vi "PixeLink OpenFocSpot.vi"(7 "Open Focal spot":path=path "G:/Développement de Programmes/Programmes/octo-labview/PixeLink - Homebrew/Data") -> ()   [LabVIEW 2014]
panel:
  in  "SOTP":bool
  out "Intensity (measured)\nx10^18 W/cm²":dbl=2.0
  out "Intensity (gaussian)\nx10^18 W/cm²":dbl=2.0
  out "Peak power (TW)":dbl=2.0
  out "FWHM y (µm)":dbl=2.0
  out "FWHM x (µm)":dbl=2.0
  in  "Transmission":dbl=0.5
  in  "Duration FWHM (fs)":dbl=4.5
  in  "Pulse Energy (mJ)":dbl=5.0
  in  "Calibration µm/px":dbl=0.5
  in  "Compute":bool
  out "Focal Spot":dbl[][](graph)
  out "Background":dbl[][](graph)
  out "ROI":dbl[][](graph)
  in  "Select Background":bool
  in  "Select ROI":bool
  # "SOTP"
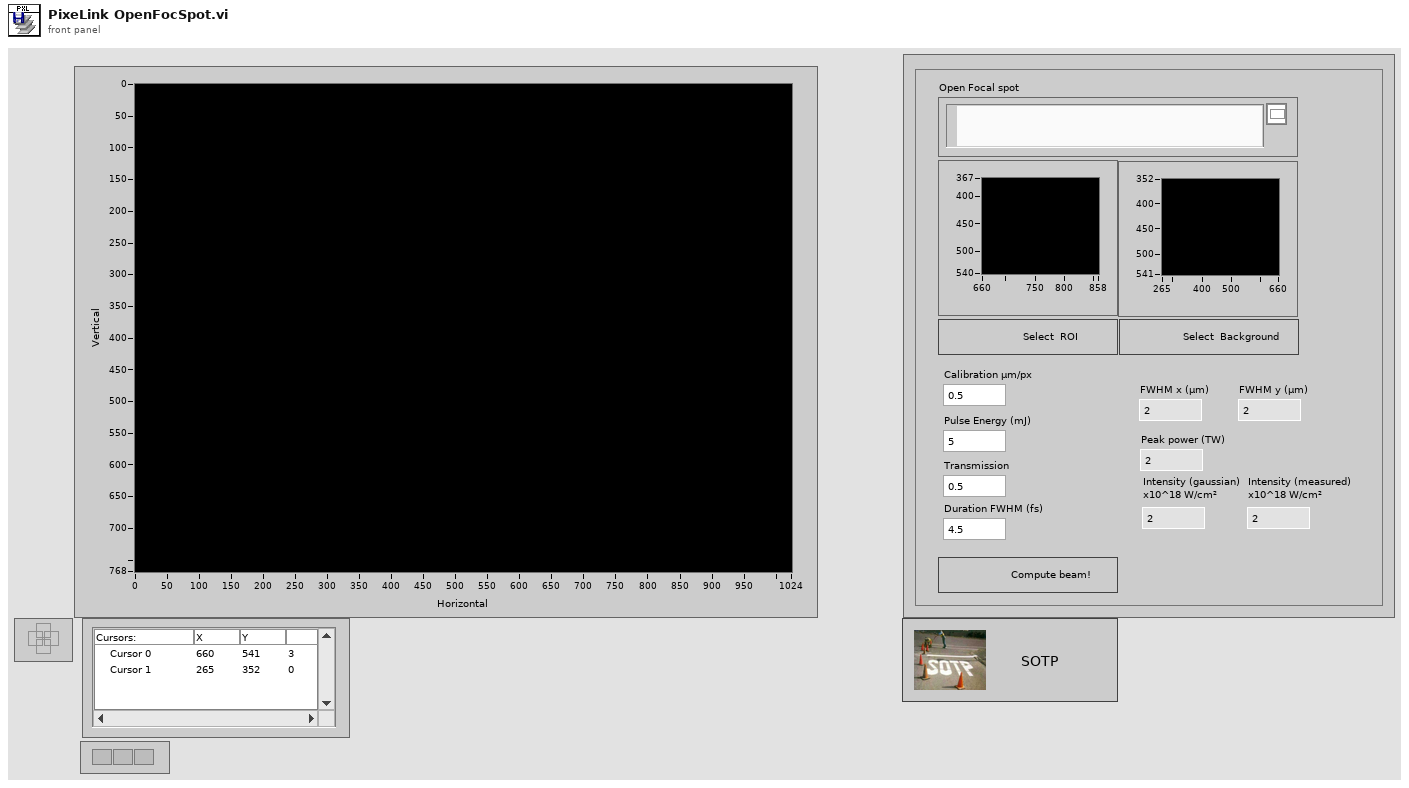
[diagram p1: front panel]
types:
  T1 = typedef "Image Type" = u32
  T2 = typedef "IMAQ Image.ctl" = refnum<image>
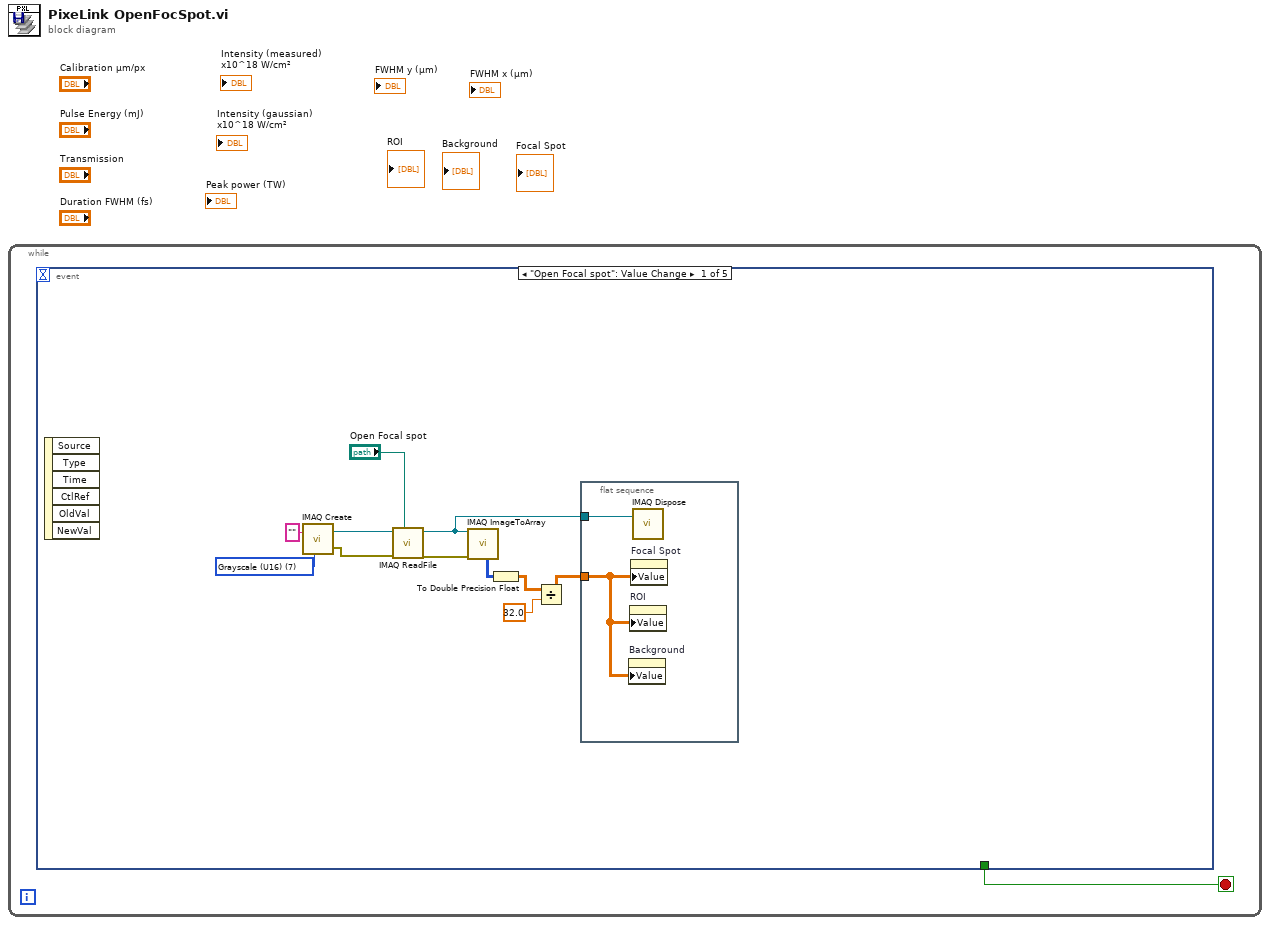
[diagram p0: block diagram]
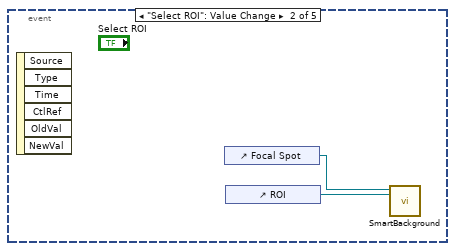
[diagram p2: hidden frame]
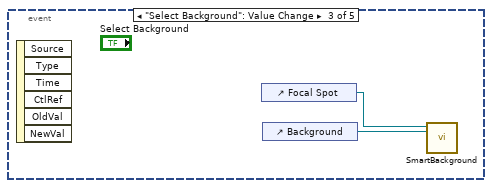
[diagram p3: hidden frame]
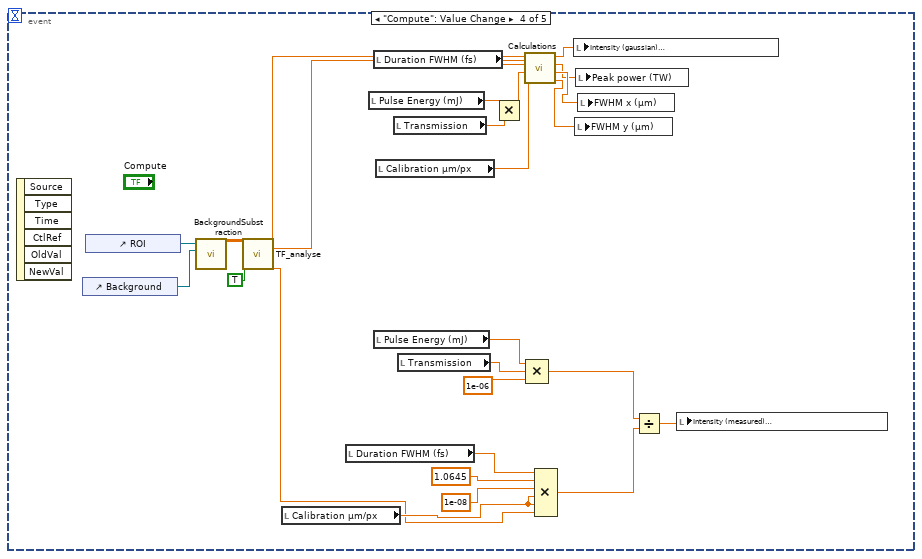
[diagram p4: hidden frame]
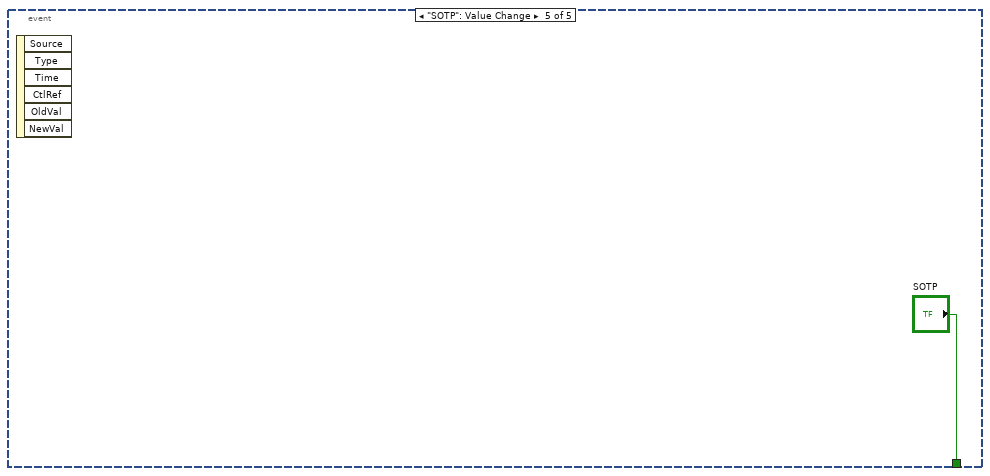
[diagram p5: hidden frame]
diagram:
  n1 = while {
    stop <- w1 stop-if-true
    n2 = event shown="[0] \"Open Focal spot\": Value Change" {
      selector: _ -> [_ _ _ _ _]
      dyn-events: _ -> [_ _ _ _ _]
      timeout: _ -> [_ _ _ _ _]
      tunnel: [_ _ _ _ "SOTP"] -> w1
      event "Open Focal spot": Value Change {
        w6 = T1 7 items=["Grayscale (U8)", "Grayscale (I16)", "Grayscale (SGL)", "Complex (CSG)", "RGB (U32)", "HSL (U32)", "RGB (U64)", "Grayscale (U16)"] ("Image Type")
        n3 = event-data() -> ()  [unwired: 1 in, 6 out]
        n4 = call "IMAQ Create"("Image Name"="", "Image Type"=w6) -> ("New Image"=w11:T2, "error out"=w9:errorcluster)  [unwired: 3 in]
        n5 = call "IMAQ ReadFile"("File Path"="Open Focal spot", "error in (no error)"=w9, "Image"=w11) -> ("error out"=w8:errorcluster, "Image Out"=w5:T2)  [unwired: 4 in, 3 out]
        n6 = call "IMAQ ImageToArray"("error in (no error)"=w8, "Image"=w5) -> ("Image Pixels (U16)"=w7:u16[][])  [unwired: 2 in, 4 out]
        n7 = To Double Precision Float(number=w7) -> (double precision float=w3:dbl[][])
        n8 = Divide(x=w3, y=32.0) -> (x/y=w4:dbl[][])
        n9 = flat-sequence {
          tunnel: w4 -> [w13]
          tunnel: w5 -> [w14]
          frame #0 {
            n10 = property on="Background" class="IntGraph (strict)"("Value"=w13) -> ()  [unwired: 2 in, 2 out]
            n11 = property on="ROI" class="IntGraph (strict)"("Value"=w13) -> ()  [unwired: 2 in, 2 out]
            n12 = property on="Focal Spot" class="IntGraph (strict)"("Value"=w13) -> ()  [unwired: 2 in, 2 out]
            n13 = call "IMAQ Dispose"("Image"=w14) -> ()  [unwired: 5 in, 1 out]
          }
        }
      }
      event "Select ROI": Value Change {
        n14 = event-data() -> ()  [unwired: 1 in, 6 out]
        n15 = control-ref of="Focal Spot"() -> (w15:refnum<vi>)
        n16 = control-ref of="ROI"() -> (w16:refnum<vi>)
        n17 = call "SmartBackground.vi"("ROI"=w16, "Input Graph"=w15) -> ()  [unwired: 10 in]
      }
      event "Select Background": Value Change {
        n18 = event-data() -> ()  [unwired: 1 in, 6 out]
        n19 = control-ref of="Focal Spot"() -> (w17:refnum<vi>)
        n20 = control-ref of="Background"() -> (w18:refnum<vi>)
        n21 = call "SmartBackground.vi"("ROI"=w18, "Input Graph"=w17) -> ()  [unwired: 10 in]
      }
      event "Compute": Value Change {
        n22 = event-data() -> ()  [unwired: 1 in, 6 out]
        n23 = control-ref of="Background"() -> (w43:refnum<vi>)
        n24 = control-ref of="ROI"() -> (w44:refnum<vi>)
        n25 = call "BackgroundSubstraction.vi"("Background Refnum"=w43, "ROI Refnum"=w44) -> ("Background Sub ROI"=w42:dbl[][])  [unwired: 9 in]
        n26 = call "TF_analyse.vi"("image 2D"=w42, "FLUENCE calculation"=TRUE) -> ("FWHM en x"=w32:dbl, "FWHM en y"=w31:dbl, "intégration totale"=w20:dbl)  [unwired: 19 in, 4 out]
        n27 = local read "Calibration µm/px"() -> (w29:dbl)
        n28 = local read "Duration FWHM (fs)"() -> (w28:dbl)
        n29 = local read "Pulse Energy (mJ)"() -> (w36:dbl)
        n30 = local read "Duration FWHM (fs)"() -> (w34:dbl)
        n31 = local read "Pulse Energy (mJ)"() -> (w27:dbl)
        n32 = local read "Calibration µm/px"() -> (w37:dbl)
        n33 = local read "Transmission"() -> (w35:dbl)
        n34 = local read "Transmission"() -> (w26:dbl)
        n35 = Multiply(x=w36, y=w35) -> (x*y=w33:dbl)
        n36 = call "Calculations.vi"("FWHM x (px)"=w32, "Calibration µm/px"=w37, "Energy in 1 Pulse (mJ)"=w33, "Pulse Duration (fs)"=w34, "FWHM y (px)"=w31) -> ("FWHM y (µm)"=w41:dbl, "FWHM x (µm)"=w40:dbl, "Peak Power (TW)"=w39:dbl, "Integral of Perfect Gaussian (x10^18 W/cm²)"=w38:dbl)  [unwired: 3 in]
        n37 = Compound Arithmetic op=MULTIPLY(w27, w26, 1e-06 ("Transmission")) -> (w22:dbl)
        n38 = Compound Arithmetic op=MULTIPLY(w28, 1.0645 ("Transmission"), 1e-08 ("Transmission"), w29, w29, w20) -> (w21:dbl)
        n39 = local write "Intensity (gaussian)\nx10^18 W/cm²"(w38) -> ()
        n40 = local write "FWHM y (µm)"(w41) -> ()
        n41 = local write "Peak power (TW)"(w39) -> ()
        n42 = local write "FWHM x (µm)"(w40) -> ()
        n43 = Divide(x=w22, y=w21) -> (x/y=w30:dbl)
        n44 = local write "Intensity (measured)\nx10^18 W/cm²"(w30) -> ()
      }
      event "SOTP": Value Change {
        n45 = event-data() -> ()  [unwired: 1 in, 6 out]
      }
    }
  }
